vi "Pockels modulation-Gen AO seq for funct img.vi"(7 "Run as sub-VI":bool, 11 "Setup/Logging queue element":T8={"Imaging Protocol"=enum."Live Imaging", "Number of Trials"=0, "Frame Size"=512, "# Averaged frames"=0, "Dwell time (us)"=0.0, "Index of Z-plane"=0, "Timelapse?"=FALSE, "Logging process is active"=FALSE, "Speed logging enabled"=FALSE, "tdms file ref"=refnum, "path"=path "", "Trial Number"=0, "Expected # points acquired"=FALSE, "Manually stopped"=FALSE, "Last trial"=FALSE, "Ch0 data"=[], "Ch1 data"=[], "Image Time"=[], "Continuous Time"=[], "Points acquired"={"Ch0 last trial"=0, "Ch1 last trial"=0, "All trials"=0}, "HW Timings File"=refnum} {"Frame Size" items=["100X100"=100, "128X128"=128, "200X200"=200, "256X256"=256, "512X512"=512, "1024x1024"=1024, "2048x2048"=2048]; "Dwell time (us)" format="%#.6g"}) -> (1 "Pockels modulation sequence":dbl[](array[numeric])=[0.0, 0.0, 0.0, 0.0, 0.0, 0.0, 0.0, 0.0, 0.0, 0.0, 0.0, 0.0, 0.0, 0.0, 0.0, 0.0, 0.0, 0.0, 0.0, 0.0, 0.0, 0.0, 0.48, 0.48, 0.48, 0.48, 0.48, 0.48, 0.0, 0.0, 0.0, 0.0, 0.0, 0.0, 0.0, 0.0, 0.0, 0.0, 0.0, 0.0, 0.0, 0.0, 0.0, 0.0, 0.0, 0.0, 0.5308080000000001, 0.5308080000000001, 0.5308080000000001, 0.5308080000000001, 0.5308080000000001, 0.5308080000000001, 0.0, 0.0, 0.0, 0.0, 0.0, 0.0, 0.0, 0.0, 0.0, 0.0, 0.0, 0.0, 0.0, 0.0, 0.0, 0.0, 0.0, 0.0, 0.0, 0.586992, 0.586992, 0.586992, 0.586992, 0.586992, 0.586992, 0.0, 0.0, 0.0, 0.0, 0.0, 0.0, 0.0, 0.0, 0.0, 0.0, 0.0, 0.0, 0.0, 0.0, 0.0, 0.0, 0.0, 0.0, 0.649124, 0.649124, 0.649124, 0.649124, 0.649124, 0.649124, 0.0, 0.0, 0.0, 0.0, 0.0, 0.0, 0.0, 0.0, 0.0, 0.0, 0.0, 0.0, 0.0, 0.0, 0.0, 0.0, 0.0, 0.0, 0.0, 0.717834, 0.717834, 0.717834, 0.717834, 0.717834, 0.717834, 0.0, 0.0, 0.0, 0.0, 0.0, 0.0, 0.0, 0.0, 0.0, 0.0, 0.0, 0.0, 0.0, 0.0, 0.0, 0.0, 0.0, 0.0, 0.793814, 0.793814, 0.793814, 0.793814, 0.793814, 0.793814, 0.0, 0.0, 0.0, 0.0, 0.0, 0.0, 0.0, 0.0, 0.0, 0.0, 0.0, 0.0, 0.0, 0.0, 0.0, 0.0, 0.0, 0.0, 0.0, 0.0, 0.0, 0.0, 0.0, 0.0, 0.0, 0.0, 0.0, 0.0, 0.0, 0.0, 0.0, 0.0, 0.0, 0.0, 0.0, 0.0, 0.0, 0.0, 0.0, 0.0, 0.0, 0.0, 0.0, 0.970756, 0.970756, 0.970756, 0.970756, 0.970756], 2 "Sampling period (us)":dbl=1e-06, 3 "Sequence length (ms)":dbl=198.0 format="%#_g ms", 4 "Sequence length (points)":i32=198 format="%.0f points")   [LabVIEW 2017]
uses:
  Typedefs/Logging queue element.ctl
  Typedefs/Imaging Protocols enum.ctl
  Typedefs/Frame Size.ctl
  Typedefs/Acquired points count.ctl
  Typedefs/Pockels-Funct acq simulation inputs cluster.ctl
  Typedefs/Controls/AOL_Globals.ctl
  Typedefs/AOL modes.ctl
  Typedefs/Plane Mode.ctl
  Typedefs/Functional Mode.ctl
  <vilib>/GPower/Comparison/Library/IsOdd/IsOddI32.vi
  <vilib>/GPower/Comparison/GPComparison.lvlib
panel:
  out "Last AOL_Globals used":T1={"Imaging Protocol"=enum."AOL Z-Stack", "Number of POI"=0, "Number of Miniscans"=0, "Number of Trials"=0, "Number of Cycles "=0, "# Averaged Frames"=0, "Laser power (%)"=0, "Pockels (V)"=0.0, "Acquisition Length (sec)"=0.0, "Fill time (us)"=0.0, "POI Dwell time (us)"=0.0, "Miniscan Dwell time per pixel (us)"=0.0, "PMT 1"=0.0, "PMT 2"=0.0, "Back Apperture (mA)"=200.0, "Frame Size"=0, "Center Frequency"=0.0, "Field of View (norm)"=0.0, "DwellTime (us)"=0.0, "Wavelength (nm)"=0.0, "Zoom"=0.0, "AOL Z"=0.0, "AOL Mode"=enum."Raster", "GridXY"=0.0, "GridZ"=0.0, "TriggerPeriod (sec)"=0.0, "Number of Pixels in Miniscan"=0, "Experiment folder path"=path "", "X centre"=0.0, "Y centre"=0.0, "Angle (degrees)"=0.0, "Plane Mode"=0, "Threshold"=[], "Regenerate Chirps"=FALSE, "Rectangle ROI length (pixels)"=0, "Rectangle ROI height (pixels)"=0, "AOD fill"=4900, "StartupDelay"=0, "Samples Wait after Trigger"=5080, "Slip Cycle"=600000, "Add Cycle"=TRUE, "Functional Mode"=enum."Point", "Z Start"=0.0, "Z Stop"=0.0, "# Planes"=0} {"Plane Mode" items=["XY Plane", "XZ Plane", "YZ Plane", "arbitraryplane"]; "Frame Size" items=["100X100"=100, "128X128"=128, "200X200"=200, "256X256"=256, "512X512"=512, "1024x1024"=1024, "2048x2048"=2048]; "Back Apperture (mA)" format="%#.6g"; "Pockels (V)" format="%#.6g"; "PMT 2" format="%#.6g"; "PMT 1" format="%#.6g"; "Angle (degrees)" format="%#.6g"; "POI Dwell time (us)" format="%#.6g"}
  in  "Temp Patch":bool=TRUE
  out "Loop":i32
  in  "Simulation inputs cluster":T7={"Dwell time (us) -Manual"=4.2, "Simulated number of POI"=80, "Bypass"=TRUE, "Pockels \"Low\" time (us)"=20.0, "AO Sample Clock Rate (samples/sec)"=1000000.0, "Control system simulated waveform"=TRUE} {"AO Sample Clock Rate (samples/sec)" format="%#_6f"; "Dwell time (us) -Manual" min=0.05 max=10.0 step=0.1 format="%#.1fus"}
  in  "Pockels turn ON at least this number of us before fill time completion":dbl=4.0 min=0.05 max=10.0 step=1.0 format="%#.1fus"
  out "Number of POI":i32=8
  out "Cursor distance (us)":dbl=2.0 format="%#_g us"
  out "AO card sampling interval (us)":dbl=1.0 format="%#_13g us"
  out "Fill time (us)":dbl=24.4 format="%#_g us"
  in  "Pockels stay ON for at least this number of us after dwell time":dbl=2.0 min=0.5 max=10.0 step=1.0 format="%#.1fus"
  out "Graph":waveform(dbl)[](graph)=[{"t0"=timestamp(0 s since 1904-01-01), "dt"=0.05, "Y"=array[4561 elements]}, {"t0"=timestamp(0 s since 1904-01-01), "dt"=1.0, "Y"=[0.0, 0.0, 0.0, 0.0, 0.0, 0.0, 0.0, 0.0, 0.0, 0.0, 0.0, 0.0, 0.0, 0.0, 0.0, 0.0, 0.0, 0.0, 0.0, 0.0, 2.0, 2.0, 2.0, 2.0, 2.0, 2.0, 2.0, 2.0, 2.0, 2.0, 2.0, 2.0, 0.0, 0.0, 0.0, 0.0, 0.0, 0.0, 0.0, 0.0, 0.0, 0.0, 0.0, 0.0, 0.0, 0.0, 0.0, 0.0, 0.0, 2.0, 2.0, 2.0, 2.0, 2.0, 2.0, 2.0, 2.0, 2.0, 2.0, 2.0, 0.0, 0.0, 0.0, 0.0, 0.0, 0.0, 0.0, 0.0, 0.0, 0.0, 0.0, 0.0, 0.0, 0.0, 0.0, 0.0, 0.0, 2.0, 2.0, 2.0, 2.0, 2.0, 2.0, 2.0, 2.0, 2.0, 2.0, 2.0, 2.0, 0.0, 0.0, 0.0, 0.0, 0.0, 0.0, 0.0, 0.0, 0.0, 0.0, 0.0, 0.0, 0.0, 0.0, 0.0, 0.0, 0.0, 2.0, 2.0, 2.0, 2.0, 2.0, 2.0, 2.0, 2.0, 2.0, 2.0, 2.0, 0.0, 0.0, 0.0, 0.0, 0.0, 0.0, 0.0, 0.0, 0.0, 0.0, 0.0, 0.0, 0.0, 0.0, 0.0, 0.0, 0.0, 2.0, 2.0, 2.0, 2.0, 2.0, 2.0, 2.0, 2.0, 2.0, 2.0, 2.0, 2.0, 0.0, 0.0, 0.0, 0.0, 0.0, 0.0, 0.0, 0.0, 0.0, 0.0, 0.0, 0.0, 0.0, 0.0, 0.0, 0.0, 0.0, 2.0, 2.0, 2.0, 2.0, 2.0, 2.0, 2.0, 2.0, 2.0, 2.0, 2.0, 0.0, 0.0, 0.0, 0.0, 0.0, 0.0, 0.0, 0.0, 0.0, 0.0, 0.0, 0.0, 0.0, 0.0, 0.0, 0.0, 0.0, 2.0, 2.0, 2.0, 2.0, 2.0, 2.0, 2.0, 2.0, 2.0, 2.0, 2.0, 2.0, 0.0, 0.0, 0.0, 0.0, 0.0, 0.0, 0.0, 0.0, 0.0, 0.0, 0.0, 0.0, 0.0, 0.0, 0.0, 0.0, 0.0, 2.0, 2.0, 2.0, 2.0, 2.0, 2.0, 2.0]}]
  # "NOTE!\nThe always-simulated \"Control System\" signal may be wrong when Movement Correction is active as it won't include the reference frame time if\nthe number of POI result in very short original cycle time."
  # "<--- The pockels is an analogue signal which takes 3us to reach its value. Using 4us here ensures that the moment when data is acquired the pockels modulation signal has already reached its nominal value."
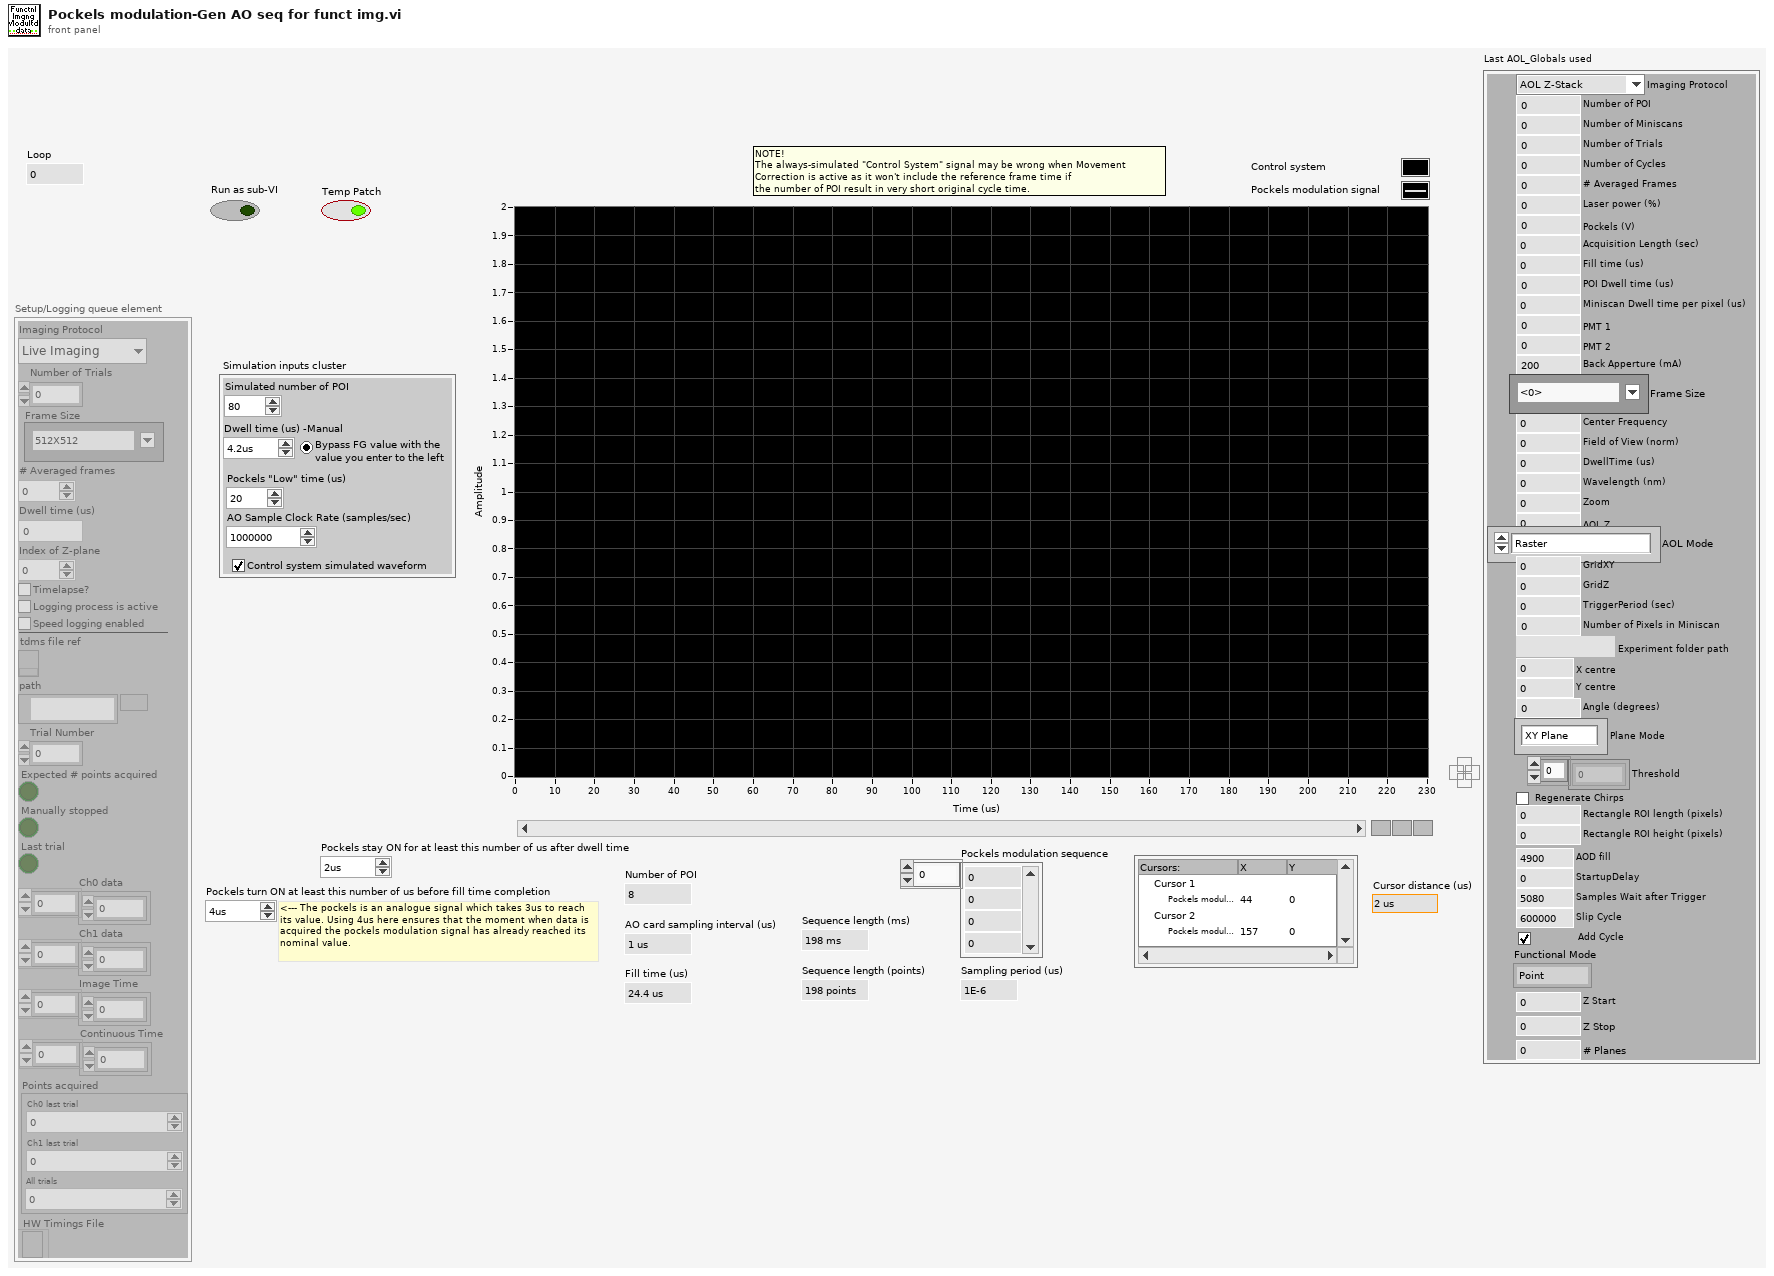
[diagram p1: front panel]
types:
  T1 = typedef "AOL_Globals.ctl" = cluster{"Imaging Protocol":T2, "Number of POI":u16, "Number of Miniscans":u16, "Number of Trials":u16, "Number of Cycles ":u64, "# Averaged Frames":u16, "Laser power (%)":u8, "Pockels (V)":dbl, "Acquisition Length (sec)":dbl, "Fill time (us)":dbl, "POI Dwell time (us)":dbl, "Miniscan Dwell time per pixel (us)":dbl, "PMT 1":dbl, "PMT 2":dbl, "Back Apperture (mA)":dbl, "Frame Size":T3, "Center Frequency":dbl, "Field of View (norm)":dbl, "DwellTime (us)":dbl, "Wavelength (nm)":dbl, "Zoom":dbl, "AOL Z":dbl, "AOL Mode":T4, "GridXY":dbl, "GridZ":dbl, "TriggerPeriod (sec)":dbl, "Number of Pixels in Miniscan":u16, "Experiment folder path":path, "X centre":dbl, "Y centre":dbl, "Angle (degrees)":dbl, "Plane Mode":T5, "Threshold":u16[], "Regenerate Chirps":bool, "Rectangle ROI length (pixels)":u16, "Rectangle ROI height (pixels)":u16, "AOD fill":u16, "StartupDelay":i32, "Samples Wait after Trigger":u16, "Slip Cycle":u32, "Add Cycle":bool, "Functional Mode":T6, "Z Start":dbl, "Z Stop":dbl, "# Planes":i32}
  T2 = typedef "Imaging Protocols enum.ctl" = enum16{"AOL Z-Stack", "Motor Z Stack", "Functional Acquisition", "Single Plane Acquisition", "Volume Acquisition", "Live Imaging", "Live Plane Imaging", "Live Volume Imaging"}
  T3 = typedef "Frame Size.ctl" = u16
  T4 = typedef "AOL modes.ctl" = enum16{"Raster", "Structural", "Pointing", "Mini Scan", "Alignment"}
  T5 = typedef "Plane Mode.ctl" = u16
  T6 = typedef "Functional Mode.ctl" = enum16{"Point", "Line", "Patch", "Plane", "Volume"}
  T7 = typedef "Pockels-Funct acq simulation inputs cluster.ctl" = cluster{"Dwell time (us) -Manual":dbl, "Simulated number of POI":i32, "Bypass":bool, "Pockels \"Low\" time (us)":dbl, "AO Sample Clock Rate (samples/sec)":dbl, "Control system simulated waveform":bool}
  T8 = typedef "Logging queue element.ctl" = cluster{"Imaging Protocol":T2, "Number of Trials":u16, "Frame Size":T3, "# Averaged frames":u16, "Dwell time (us)":dbl, "Index of Z-plane":i32, "Timelapse?":bool, "Logging process is active":bool, "Speed logging enabled":bool, "tdms file ref":refnum<k34>, "path":path, "Trial Number":i32, "Expected # points acquired":bool, "Manually stopped":bool, "Last trial":bool, "Ch0 data":u32[], "Ch1 data":u32[], "Image Time":u64[], "Continuous Time":u64[], "Points acquired":T9, "HW Timings File":refnum<file>}
  T9 = typedef "Acquired points count.ctl" = cluster{"Ch0 last trial":u64, "Ch1 last trial":u64, "All trials":u64}
  T10 = typedef "ROI parameters data type.ctl" = cluster{"ROI index":dbl, "ROI ID":dbl, "ROI Time (ns)":dbl, "Pixels in ROI":dbl, "X start":dbl, "Y start":dbl, "Z start":dbl, "X stop":dbl, "Y stop":dbl, "Z stop":dbl, "Angle (deg)":dbl, "Composite ID":dbl, "Number of lines":dbl, "Frame Size":dbl, "Zoom":dbl, "Laser Power (%)":dbl, "ROI group ID":dbl, "Z Plane Idx":i32[], "Z Plane codes":i32[]}
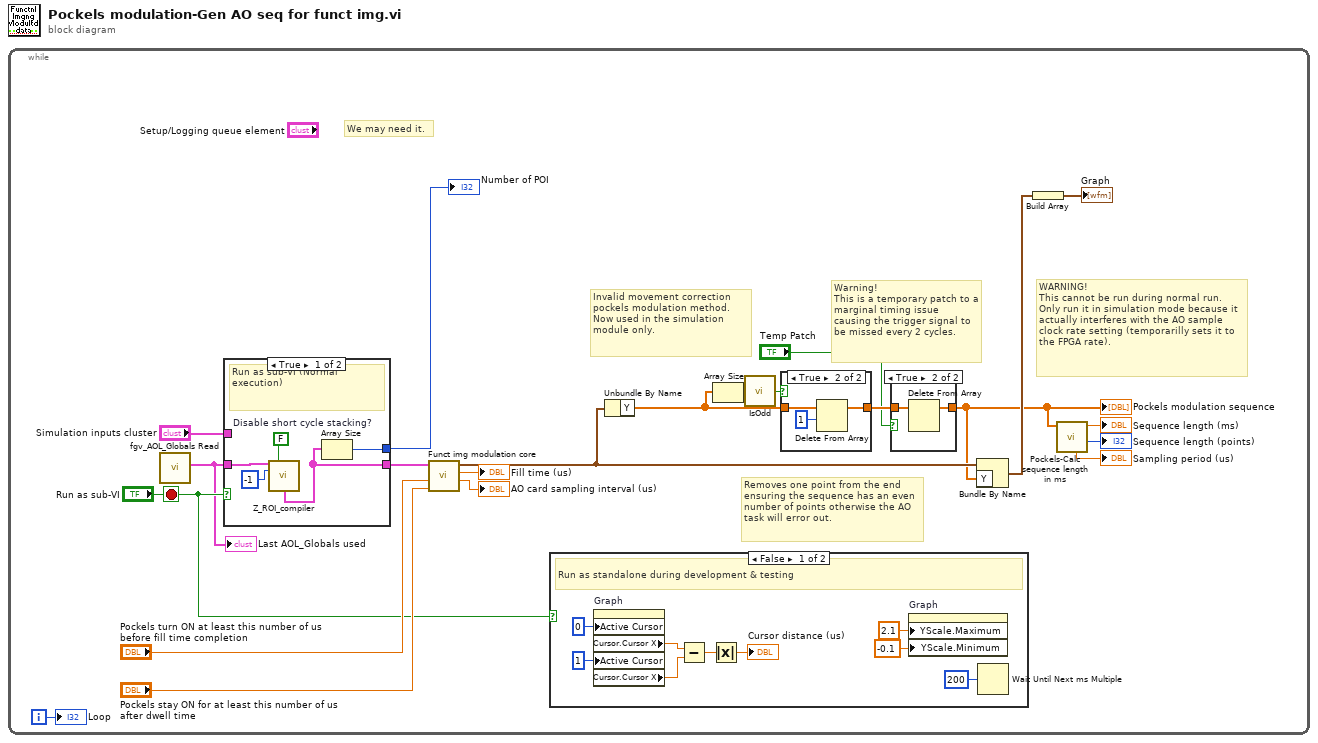
[diagram p0: block diagram]
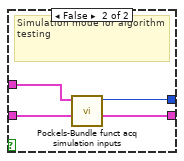
[diagram p3: hidden frame]
diagram:
  n1 = while {
    i -> [w6]
    stop <- "Run as sub-VI" stop-if-true
    # "Warning!\nThis is a temporary patch to a marginal timing issue \ncausing the trigger signal to be missed every 2 cycles."
    # "WARNING!\nThis cannot be run during normal run. Only run it in simulation mode because it actually interferes with the AO sample clock rate setting (temporarilly sets it to the FPGA rate)."
    # "Invalid movement correction pockels modulation method.\nNow used in the simulation module only."
    # "We may need it."
    # "Removes one point from the end ensuring the sequence has an even number of points otherwise the AO task will error out."
    n2 = call "fgv_AOL_Globals Read.vi"() -> ("AOL_Globals"=w2:T1)  [unwired: 9 in, 2 out]
    "Last AOL_Globals used" <- w2
    n3 = case shown="True" "Run as sub-VI" {
      tunnel: [w27 w33] -> w16
      tunnel: [w30 w34] -> w4
      tunnel: w2 -> [w29 w32]
      tunnel: "Simulation inputs cluster" -> [_ w31]
      frame True {
        w26 = FALSE  # Disable short cycle stacking?
        # "Run as sub-VI (Normal execution)"
        n4 = call "Z_ROI_compiler.vi"("AOL_Globals"=w29, "dISABLE"=w26, "Acquired z-plane index / volume index"=-1) -> ("ROI Attributes (broken down to miniscans)"=w27:T10[])  [unwired: 5 in, 7 out]
        n5 = Array Size(array=w27) -> (size(s)=w30:i32)
      }
      frame False {
        # "Simulation mode for algorithm testing"
        n6 = call "Pockels-Bundle funct acq simulation inputs.vi"("AOL_Globals"=w32, "Simulation inputs cluster"=w31) -> ("Array"=w33:T10[], "Simulated number of POI"=w34:i32)  [unwired: 8 in]
      }
    }
    "Number of POI" <- w4
    n7 = call "Funct img modulation core.vi"("Pockels stay ON for at least this number of us after dwell time"="Pockels stay ON for at least this number of us after dwell time", "Pockels turn ON at least this number of us before fill time completion"="Pockels turn ON at least this number of us before fill time completion", "ROI setup"=w16) -> ("AO card sampling interval (us)"=→"AO card sampling interval (us)":dbl, "Fill time (us)"=→"Fill time (us)":dbl, "waveform out"=w13:waveform(dbl))  [unwired: 5 in, 1 out]
    n8 = case shown="False" "Run as sub-VI" {
      frame False {
        # "Run as standalone during development & testing"
        n9 = property on="Graph" class="WFGraph (strict)"("Active Cursor"=u32 0, "Active Cursor"=u32 1) -> ("Cursor.Cursor X"=w44:dbl, "Cursor.Cursor X"=w43:dbl)  [unwired: 2 in, 2 out]
        n10 = Subtract(x=w44, y=w43) -> (x-y=w42:dbl)
        n11 = Absolute Value(x=w42) -> (abs(x)=→"Cursor distance (us)":dbl)
        n12 = property on="Graph" class="WFGraph (strict)"("YScale.Maximum"=2.1 ("Y Scale.Range:Maximum"), "YScale.Minimum"=-0.1 ("Y Scale.Range:Minimum")) -> ()  [unwired: 2 in, 2 out]
        n13 = Wait Until Next ms Multiple(millisecond multiple=u32 200) -> ()  [unwired: 1 out]
      }
      frame True {
        # "Run as sub-VI"
      }
    }
    n14 = Unbundle By Name(w13) -> ("Y"=w18:dbl[])
    n15 = Array Size(array=w18) -> (size(s)=w22:i32)
    n16 = call-poly <vilib>:"IsOdd.vi"("x"=w22) -> ("Odd?"=w21:bool)  [unwired: 4 in]
    n17 = case shown="True" w21 {
      tunnel: w18 -> [w35 w38]
      tunnel: [w35 w37] -> w20
      frame False {
      }
      frame True {
        n18 = Delete From Array(array=w38, length=1) -> (array with subset deleted=w37:dbl[])  [unwired: 1 in, 1 out]
      }
    }
    n19 = case shown="True" "Temp Patch" {
      tunnel: w20 -> [w23 w25]
      tunnel: [w23 w24] -> w10
      frame False {
      }
      frame True {
        n20 = Delete From Array(array=w25) -> (array with subset deleted=w24:dbl[])  [unwired: 2 in, 1 out]
      }
    }
    "Pockels modulation sequence" <- w10
    n21 = Bundle By Name(cluster=w13, "Y"=w10) -> (w19:waveform(dbl))
    n22 = Build Array(w19) -> (→"Graph":waveform(dbl)[])
    n23 = call "Pockels-Calc sequence length in ms.vi"("Pockels modulation sequence in"=w10) -> ("Sequence length (points)"=→"Sequence length (points)":i32, "Sequence length (ms)"=→"Sequence length (ms)":dbl, "Sampling period (us)"=→"Sampling period (us)":dbl)  [unwired: 8 in]
    "Loop" <- w6
  }
